vi "State Machine.vi"(8 "error in (no error)":errorcluster) -> (0 "error out":errorcluster)   [LabVIEW 2018]
uses:
  State Machine/State Machine.lvclass
  State Machine/State Machine.lvclass/State Machine.ctl
  <vilib>/addons/_JKI Toolkits/Caraya/classes/Test/Test.lvclass
  <vilib>/addons/_JKI Toolkits/Caraya/classes/Assert/Assert.lvclass
panel:
  in  "State Machine in 2":refnum<class "State Machine.lvclass">
  in  "State Machine in":refnum<class "State Machine.lvclass">
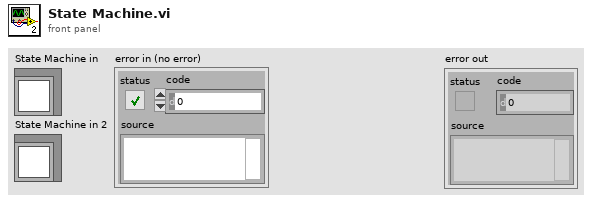
[diagram p1: front panel]
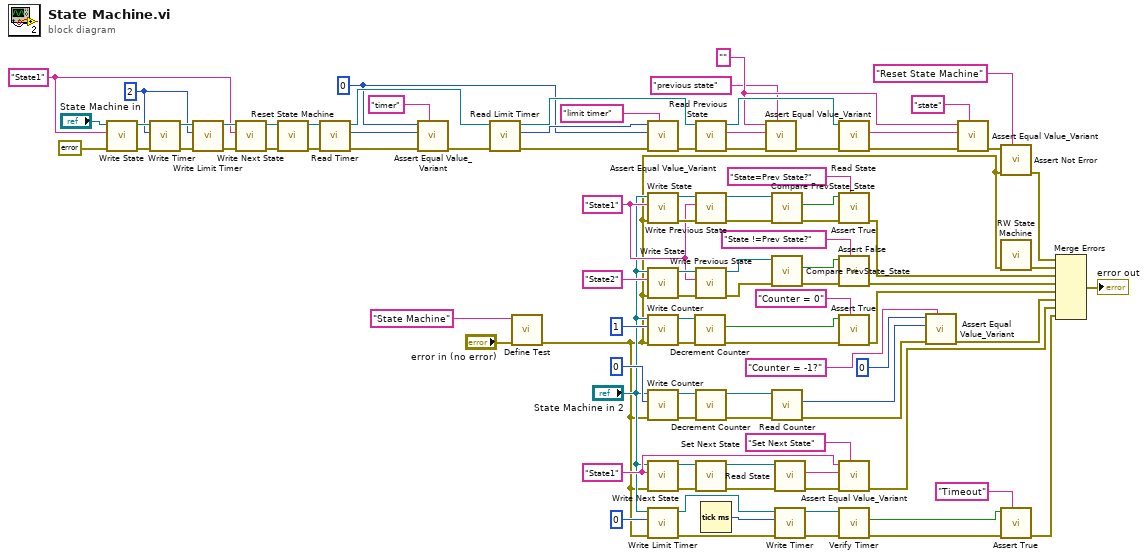
[diagram p0: block diagram]
diagram:
  w20 = "State1" ("Label (VI Title)")
  w29 = "" ("State")
  w36 = u16 0 ("Counter")
  w52 = u16 2 ("Counter")
  w53 = "State1" ("Label (VI Title)")
  w77 = "State1" ("Label (VI Title)")
  n1 = call-dynamic "Write State.vi"("error in (no error)"=errorcluster {"status"=FALSE, "code"=0, "source"=""}, "State"=w53, "State Machine in"="State Machine in") -> ("error out"=w57:errorcluster, "State Machine out"=w56:refnum<class "State Machine.lvclass">)  [unwired: 7 in]
  n2 = call "Write Timer.vi"("error in (no error)"=w57, "Timer"=w52, "State Machine in"=w56) -> ("error out"=w58:errorcluster, "State Machine out"=w55:refnum<class "State Machine.lvclass">)  [unwired: 7 in]
  n3 = call "Write Limit Timer.vi"("error in (no error)"=w58, "Limit Timer"=w52, "State Machine in"=w55) -> ("error out"=w59:errorcluster, "State Machine out"=w54:refnum<class "State Machine.lvclass">)  [unwired: 7 in]
  n4 = call "Write Next State.vi"("error in (no error)"=w59, "Next State"=w53, "State Machine in"=w54) -> ("error out"=w51:errorcluster, "State Machine out"=w50:refnum<class "State Machine.lvclass">)  [unwired: 7 in]
  n5 = call "Reset State Machine.vi"("error in (no error)"=w51, "State Machine in"=w50) -> ("error out"=w45:errorcluster, "State Machine out"=w46:refnum<class "State Machine.lvclass">)  [unwired: 8 in]
  n6 = call "Read Timer.vi"("error in (no error)"=w45, "State Machine in"=w46) -> ("error out"=w44:errorcluster, "Timer"=w42:u32, "State Machine out"=w47:refnum<class "State Machine.lvclass">)  [unwired: 7 in]
  n7 = call <vilib>:"Assert Equal Value_Variant.vi"("Label"="timer", "error in (no error)"=w44, "Actual"=w42, "Expected"=w36) -> ("error out"=w43:errorcluster)  [unwired: 6 in, 1 out]
  n8 = call "Read Limit Timer.vi"("error in (no error)"=w43, "State Machine in"=w47) -> ("error out"=w38:errorcluster, "Limit Timer"=w37:u32, "State Machine out"=w48:refnum<class "State Machine.lvclass">)  [unwired: 7 in]
  n9 = call <vilib>:"Define Test.vi"("error in (no error)"="error in (no error)", "Label (VI Title)"="State Machine") -> ("error out"=w15:errorcluster)  [unwired: 8 in, 1 out]
  n10 = call <vilib>:"Assert Equal Value_Variant.vi"("Label"="limit timer", "error in (no error)"=w38, "Actual"=w36, "Expected"=w37) -> ("error out"=w39:errorcluster)  [unwired: 6 in, 1 out]
  n11 = call-dynamic "Write State.vi"("error in (no error)"=w15, "State"=w77, "State Machine in"="State Machine in 2") -> ("error out"=w94:errorcluster, "State Machine out"=w93:refnum<class "State Machine.lvclass">)  [unwired: 7 in]
  n12 = call-dynamic "Write State.vi"("error in (no error)"=w15, "State"="State2" ("Label (VI Title)"), "State Machine in"="State Machine in 2") -> ("error out"=w79:errorcluster, "State Machine out"=w80:refnum<class "State Machine.lvclass">)  [unwired: 7 in]
  n13 = call "Write Counter.vi"("error in (no error)"=w15, "Counter"=u16 1, "State Machine in"="State Machine in 2") -> ("error out"=w74:errorcluster, "State Machine out"=w73:refnum<class "State Machine.lvclass">)  [unwired: 7 in]
  n14 = call "Write Counter.vi"("error in (no error)"=w15, "Counter"=u16 0, "State Machine in"="State Machine in 2") -> ("error out"=w67:errorcluster, "State Machine out"=w68:refnum<class "State Machine.lvclass">)  [unwired: 7 in]
  n15 = call "Write Next State.vi"("error in (no error)"=w15, "Next State"=w20, "State Machine in"="State Machine in 2") -> ("error out"=w27:errorcluster, "State Machine out"=w26:refnum<class "State Machine.lvclass">)  [unwired: 7 in]
  n16 = call "Write Limit Timer.vi"("error in (no error)"=w15, "Limit Timer"=u32 0, "State Machine in"="State Machine in 2") -> ("error out"=w8:errorcluster, "State Machine out"=w7:refnum<class "State Machine.lvclass">)  [unwired: 7 in]
  n17 = call "Decrement Counter.vi"("error in (no error)"=w74, "State Machine in"=w73) -> ("error out"=w72:errorcluster, "counter = zero"=w69:bool)  [unwired: 7 in, 1 out]
  n18 = call-dynamic "Read Previous State.vi"("error in (no error)"=w39, "State Machine in"=w48) -> ("error out"=w35:errorcluster, "Previous State"=w30:string, "State Machine out"=w49:refnum<class "State Machine.lvclass">)  [unwired: 7 in]
  n19 = call-dynamic "Write Previous State.vi"("error in (no error)"=w94, "Previous State"=w77, "State Machine in"=w93) -> ("error out"=w95:errorcluster, "State Machine out"=w92:refnum<class "State Machine.lvclass">)  [unwired: 7 in]
  n20 = call-dynamic "Write Previous State.vi"("error in (no error)"=w79, "Previous State"=w77, "State Machine in"=w80) -> ("error out"=w78:errorcluster, "State Machine out"=w81:refnum<class "State Machine.lvclass">)  [unwired: 7 in]
  n21 = call "Decrement Counter.vi"("error in (no error)"=w67, "State Machine in"=w68) -> ("error out"=w65:errorcluster, "State Machine out"=w64:refnum<class "State Machine.lvclass">)  [unwired: 7 in, 1 out]
  n22 = call "Set Next State.vi"("error in (no error)"=w27, "State Machine in"=w26) -> ("error out"=w24:errorcluster, "State Machine out"=w23:refnum<class "State Machine.lvclass">)  [unwired: 8 in]
  n23 = Tick Count (ms)() -> (millisecond timer value=w6:u32)
  n24 = call <vilib>:"Assert Equal Value_Variant.vi"("Label"="previous state", "error in (no error)"=w35, "Actual"=w30, "Expected"=w29) -> ("error out"=w34:errorcluster)  [unwired: 6 in, 1 out]
  n25 = call "Compare PrevState_State.vi"("error in (no error)"=w95, "State Machine in"=w92) -> ("error out"=w89:errorcluster, "prev = state ?"=w87:bool)  [unwired: 7 in, 1 out]
  n26 = call "Compare PrevState_State.vi"("error in (no error)"=w78, "State Machine in"=w81) -> ("error out"=w82:errorcluster, "prev = state ?"=w84:bool)  [unwired: 7 in, 1 out]
  n27 = call "Read Counter.vi"("error in (no error)"=w65, "State Machine in"=w64) -> ("error out"=w62:errorcluster, "Counter"=w5:u16)  [unwired: 7 in, 1 out]
  n28 = call-dynamic "Read State.vi"("error in (no error)"=w24, "State Machine in"=w23) -> ("error out"=w22:errorcluster, "State"=w21:string)  [unwired: 7 in, 1 out]
  n29 = call "Write Timer.vi"("error in (no error)"=w8, "Timer"=w6, "State Machine in"=w7) -> ("error out"=w10:errorcluster, "State Machine out"=w9:refnum<class "State Machine.lvclass">)  [unwired: 7 in]
  n30 = call-dynamic "Read State.vi"("error in (no error)"=w34, "State Machine in"=w49) -> ("error out"=w33:errorcluster, "State"=w31:string)  [unwired: 7 in, 1 out]
  n31 = call <vilib>:"Assert True.vi"("Label"="State=Prev State?", "error in (no error)"=w89, "True?"=w87) -> ("error out"=w88:errorcluster)  [unwired: 7 in, 1 out]
  n32 = call <vilib>:"Assert False.vi"("Label"="State !=Prev State?", "error in (no error)"=w82, "False?"=w84) -> ("error out"=w76:errorcluster)  [unwired: 7 in, 1 out]
  n33 = call <vilib>:"Assert True.vi"("Label"="Counter = 0", "error in (no error)"=w72, "True?"=w69) -> ("error out"=w70:errorcluster)  [unwired: 7 in, 1 out]
  n34 = call <vilib>:"Assert Equal Value_Variant.vi"("Label"="Set Next State", "error in (no error)"=w22, "Actual"=w21, "Expected"=w20) -> ("error out"=w18:errorcluster)  [unwired: 6 in, 1 out]
  n35 = call "Verify Timer.vi"("error in (no error)"=w10, "State Machine in"=w9) -> ("error out"=w14:errorcluster, "time out"=w11:bool)  [unwired: 7 in, 1 out]
  n36 = call <vilib>:"Assert Equal Value_Variant.vi"("Label"="Counter = -1?", "error in (no error)"=w62, "Actual"=w5, "Expected"=u16 0 ("Counter")) -> ("error out"=w61:errorcluster)  [unwired: 6 in, 1 out]
  n37 = call <vilib>:"Assert Equal Value_Variant.vi"("Label"="state", "error in (no error)"=w33, "Actual"=w31, "Expected"=w29) -> ("error out"=w32:errorcluster)  [unwired: 6 in, 1 out]
  n38 = call <vilib>:"Assert Not Error.vi"("Label"="Reset State Machine", "error in (no error)"=w15, "Not Error?"=w32) -> ("error out"=w41:errorcluster)  [unwired: 7 in, 1 out]
  n39 = call "RW State Machine.vi"("error in (no error)"=w15) -> ("error out"=w91:errorcluster)  [unwired: 10 in]
  n40 = call <vilib>:"Assert True.vi"("Label"="Timeout", "error in (no error)"=w14, "True?"=w11) -> ("error out"=w13:errorcluster)  [unwired: 7 in, 1 out]
  n41 = Merge Errors(w41, w91, w88, w76, w70, w61, w18, w13) -> (→"error out":errorcluster)
